vi "CanGrabberControl.vi"(8 "error in":errorcluster) -> ()   [LabVIEW 2014]
uses:
  Utilities/CanGrabberSetpoint.vi
panel:
  in  "AllowedEncoderError":dbl=25.0 format="%#_13g"
  in  "AllowedTimeDeviation":dbl=2.4 format="%#_13g"
  out "TimeOfLastChange":timestamp=timestamp(3512669090.758719 s since 1904-01-01)
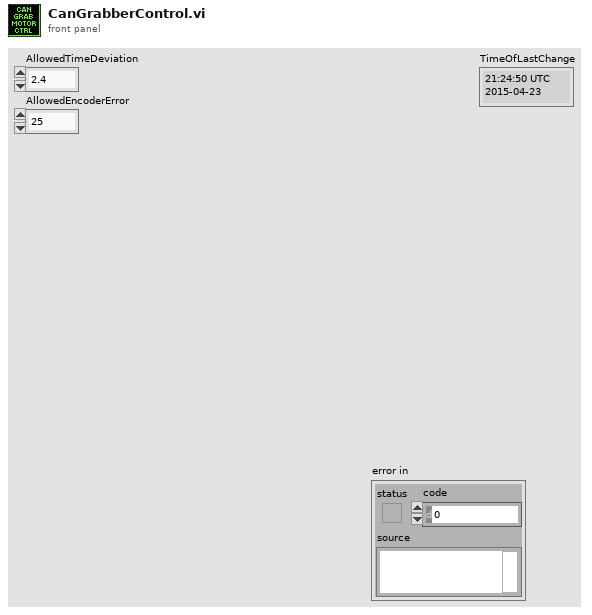
[diagram p1: front panel]
types:
  T1 = typedef "WPI_MotorControlDeviceRef.ctl" = cluster{"DeviceStatus":errorcluster, "Type":T2, "PWM":cluster{"Controller":T3, "PWM Channel":T4, "DeadBand":T5}, "CAN":cluster{"Device Number":u8, "Control Mode":T6, "Semaphore":T7, "Max Vout":dbl, "TalonSRX Control Mode":T8}, "Invert":bool, "TransformRef":T9, "InvTransformRef":T9}
  T2 = typedef "WPI_MotorControlType.ctl" = enum16{"PWM", "CAN", "CANTalonSRX"}
  T3 = typedef "FPGA_TypedefDigitalModule.ctl" = enum16{"Controller 1"}
  T4 = typedef "FPGA_DIOPWMChannel.ctl" = enum8{"PWM 0", "PWM 1", "PWM 2", "PWM 3", "PWM 4", "PWM 5", "PWM 6", "PWM 7", "PWM 8", "PWM 9", "PWM MXP 0", "PWM MXP 1", "PWM MXP 2", "PWM MXP 3", "PWM MXP 4", "PWM MXP 5", "PWM MXP 6", "PWM MXP 7", "PWM MXP 8", "PWM MXP 9", "Invalid"}
  T5 = typedef "WPI_PWMDeadband.ctl" = cluster{"Name":string, "maxPositivePwm":i32, "minPositivePwm":i32, "centerPwm":i32, "maxNegativePwm":i32, "minNegativePwm":i32, "angularRange":u16}
  T6 = typedef "WPI_CANJaguar_ControlMode.ctl" = enum8{"Percent VBus", "Current", "Speed", "Position", "Voltage"}
  T7 = typedef "Semaphore RefNum" = refnum<k1>
  T8 = typedef "WPI_CANTalonSRX_APIControlMode.ctl" = enum8{"Percent VBus", "Speed", "Position", "Slave", "Unchanged / Invalid"}
  T9 = typedef "WPI_PWMTransform_ConPane.ctl" = refnum<vi>
  T10 = typedef "WPI_CANTalonSRX_GlobalStatus.ctl" = cluster{"Applied Throttle":dbl, "Module Enabled":bool, "CAN Error":errorcluster, "Closed Loop Error":dbl, "Forward Limit Switch Closed":bool, "Reverse Limit Switch Closed":bool, "Sensor Position":dbl, "Sensor Velocity":dbl, "Current":dbl, "Sticky Fault - Over Temp":bool, "Sticky Fault - Under Voltage":bool, "Sticky Fault - Forward Limit":bool, "Sticky Fault - Reverse Limit":bool, "Sticky Fault - Forward Soft Limit":bool, "Sticky Fault - Reverse Soft Limit":bool, "Brake is Enabled":bool, "Encoder Position":dbl, "Encoder Velocity":dbl, "Encoder Index Count":dbl, "Encoder A Pin State":bool, "Encoder B Pin State":bool, "Encoder Index Pin State":bool, "Analog In":dbl, "Analog In Velocity":dbl, "Temperature (C)":dbl, "Battery Voltage":dbl}
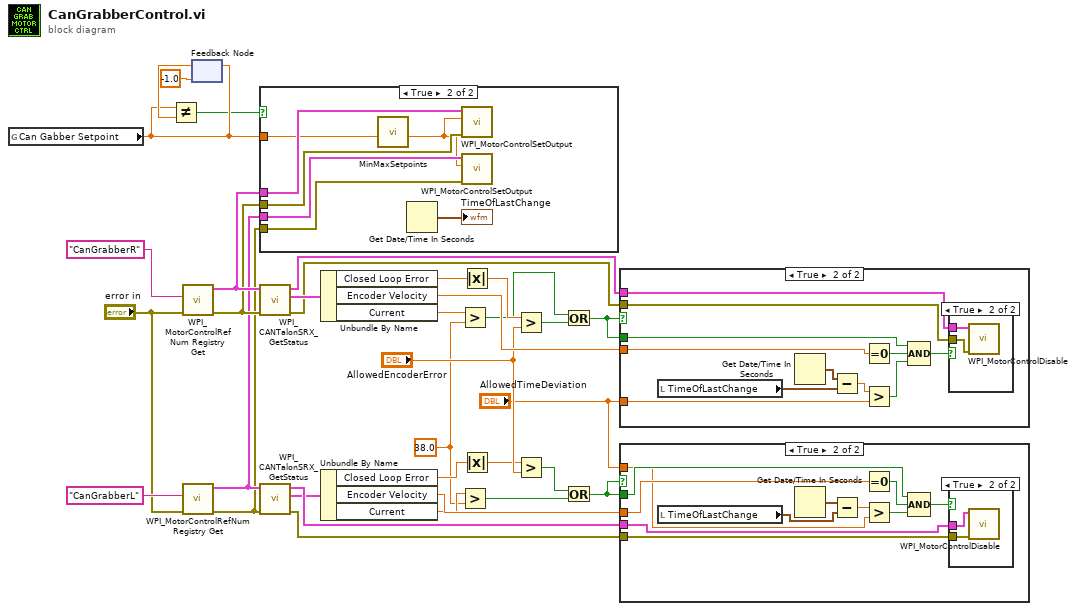
[diagram p0: block diagram]
diagram:
  w4 = 38.0 ("y")
  n1 = global read "CanGrabberSetpoint.vi" "Can Gabber Setpoint"() -> (w29:dbl)
  n2 = call <vilib>:"WPI_MotorControlRefNum Registry Get.vi"("error in (no error)"="error in", "refnum name"="CanGrabberR") -> ("error out"=w26:errorcluster, "MotorControlDevRef"=w27:T1)  [unwired: 8 in]
  n3 = call <vilib>:"WPI_MotorControlRefNum Registry Get.vi"("error in (no error)"="error in", "refnum name"="CanGrabberL") -> ("error out"=w14:errorcluster, "MotorControlDevRef"=w15:T1)  [unwired: 8 in]
  n4 = feedback #1(-1.0 ("LiftSetpoint")) -> (w34:dbl)
  n5 = Not Equal?(x=w29, y=w34) -> (x != y?=w24:bool)
  n6 = feedback-in #1(w29) -> ()
  n7 = case shown="True" w24 {
    tunnel: w29 -> [_ w37]
    tunnel: w15 -> [_ w41]
    tunnel: w14 -> [_ w40]
    tunnel: w27 -> [_ w39]
    tunnel: w26 -> [_ w38]
    frame False {
    }
    frame True {
      n8 = call "MinMaxSetpoints.vi"("CanGrabberIn"=w37) -> ("CanGrabberOut"=w36:dbl)  [unwired: 8 in, 2 out]
      n9 = Get Date/Time In Seconds() -> (seconds since 1Jan1904=→"TimeOfLastChange":timestamp)
      n10 = call <vilib>:"WPI_MotorControlSetOutput.vi"("error in (no error)"=w38, "Output"=w36, "MotorControlDevRef"=w39) -> ()  [unwired: 6 in, 3 out]
      n11 = call <vilib>:"WPI_MotorControlSetOutput.vi"("error in (no error)"=w40, "Output"=w36, "MotorControlDevRef"=w41) -> ()  [unwired: 6 in, 3 out]
    }
  }
  n12 = call <vilib>:"WPI_CANTalonSRX_GetStatus.vi"("error in (no error)"=w26, "CAN Talon SRX Ref"=w27) -> ("error out"=w21:errorcluster, "Talon SRX Status"=w28:T10, "CAN Talon SRX Ref Out"=w22:T1)  [unwired: 7 in]
  n13 = call <vilib>:"WPI_CANTalonSRX_GetStatus.vi"("error in (no error)"=w14, "CAN Talon SRX Ref"=w15) -> ("error out"=w20:errorcluster, "Talon SRX Status"=w16:T10, "CAN Talon SRX Ref Out"=w19:T1)  [unwired: 7 in]
  n14 = Unbundle By Name(w28) -> ("Closed Loop Error"=w25:dbl, "Encoder Velocity"=w23:dbl, "Current"=w9:dbl)
  n15 = Unbundle By Name(w16) -> ("Closed Loop Error"=w17:dbl, "Encoder Velocity"=w18:dbl, "Current"=w5:dbl)
  n16 = Greater?(x=w9, y=w4) -> (0:w8:bool)
  n17 = Greater?(x=w5, y=w4) -> (0:w3:bool)
  n18 = Absolute Value(x=w25) -> (abs(x)=w11:dbl)
  n19 = Absolute Value(x=w17) -> (abs(x)=w10:dbl)
  n20 = Greater?(x=w11, y="AllowedEncoderError") -> (0:w7:bool)
  n21 = Greater?(x=w10, y="AllowedEncoderError") -> (0:w2:bool)
  n22 = Or(x=w8, y=w7) -> (x .or. y?=w6:bool)
  n23 = Or(x=w2, y=w3) -> (x .or. y?=w1:bool)
  n24 = case shown="True" w6 {
    tunnel: w6 -> [_ w46]
    tunnel: w23 -> [_ w52]
    tunnel: w22 -> [_ w51]
    tunnel: w21 -> [_ w50]
    tunnel: "AllowedTimeDeviation" -> [_ w42]
    frame False {
    }
    frame True {
      n25 = local read "TimeOfLastChange"() -> (w48:timestamp)
      n26 = Get Date/Time In Seconds() -> (seconds since 1Jan1904=w49:timestamp)
      n27 = Subtract(x=w49, y=w48) -> (x-y=w47:dbl)
      n28 = Equal To 0?(x=w52) -> (x = 0?=w45:bool)
      n29 = Greater?(x=w47, y=w42) -> (0:w44:bool)
      n30 = Compound Arithmetic op=AND(w46, w45, w44) -> (w43:bool)
      n31 = case shown="True" w43 {
        tunnel: w51 -> [_ w54]
        tunnel: w50 -> [_ w53]
        frame False {
        }
        frame True {
          n32 = call <vilib>:"WPI_MotorControlDisable.vi"("error in (no error)"=w53, "MotorControlDevRef"=w54) -> ()  [unwired: 8 in, 2 out]
        }
      }
    }
  }
  n33 = case shown="True" w1 {
    tunnel: w1 -> [_ w59]
    tunnel: w18 -> [_ w65]
    tunnel: w19 -> [_ w64]
    tunnel: w20 -> [_ w63]
    tunnel: "AllowedTimeDeviation" -> [_ w55]
    frame False {
    }
    frame True {
      n34 = local read "TimeOfLastChange"() -> (w61:timestamp)
      n35 = Get Date/Time In Seconds() -> (seconds since 1Jan1904=w62:timestamp)
      n36 = Subtract(x=w62, y=w61) -> (x-y=w60:dbl)
      n37 = Equal To 0?(x=w65) -> (x = 0?=w58:bool)
      n38 = Greater?(x=w60, y=w55) -> (0:w57:bool)
      n39 = Compound Arithmetic op=AND(w59, w58, w57) -> (w56:bool)
      n40 = case shown="True" w56 {
        tunnel: w64 -> [_ w67]
        tunnel: w63 -> [_ w66]
        frame False {
        }
        frame True {
          n41 = call <vilib>:"WPI_MotorControlDisable.vi"("error in (no error)"=w66, "MotorControlDevRef"=w67) -> ()  [unwired: 8 in, 2 out]
        }
      }
    }
  }
